vi "Update Bind Method Constants.vi"(7 "RPC Method Parameters":T1[](array[typedef]), 8 "error in (no error)":errorcluster, 10 "RPC Method Name":string, 11 "VI in":refnum<vi>) -> (0 "error out":errorcluster, 3 "VI out":refnum<vi>)   [LabVIEW 2019, in "gRPC Scripting Tools.lvlib"]
uses:
  gRPC Scripting Tools.lvlib
  TypeDefs/RPC Method Parameters.ctl
  <vilib>/Utility/traverseref.llb/TRef TravTarget.ctl
  <vilib>/Utility/traverseref.llb/VI Scripting - Traverse.lvlib
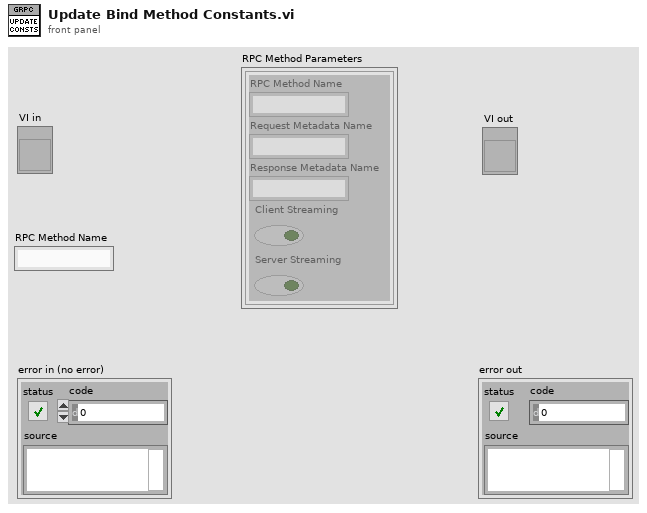
[diagram p1: front panel]
types:
  T1 = typedef "gRPC Scripting Tools.lvlib/RPC Method Parameters.ctl" = cluster{"RPC Method Name":string, "Request Metadata Name":string, "Response Metadata Name":string, "Client Streaming":bool, "Server Streaming":bool}
  T2 = typedef "TRef TravTarget.ctl" = enum16{"FP", "BD", "Other"}
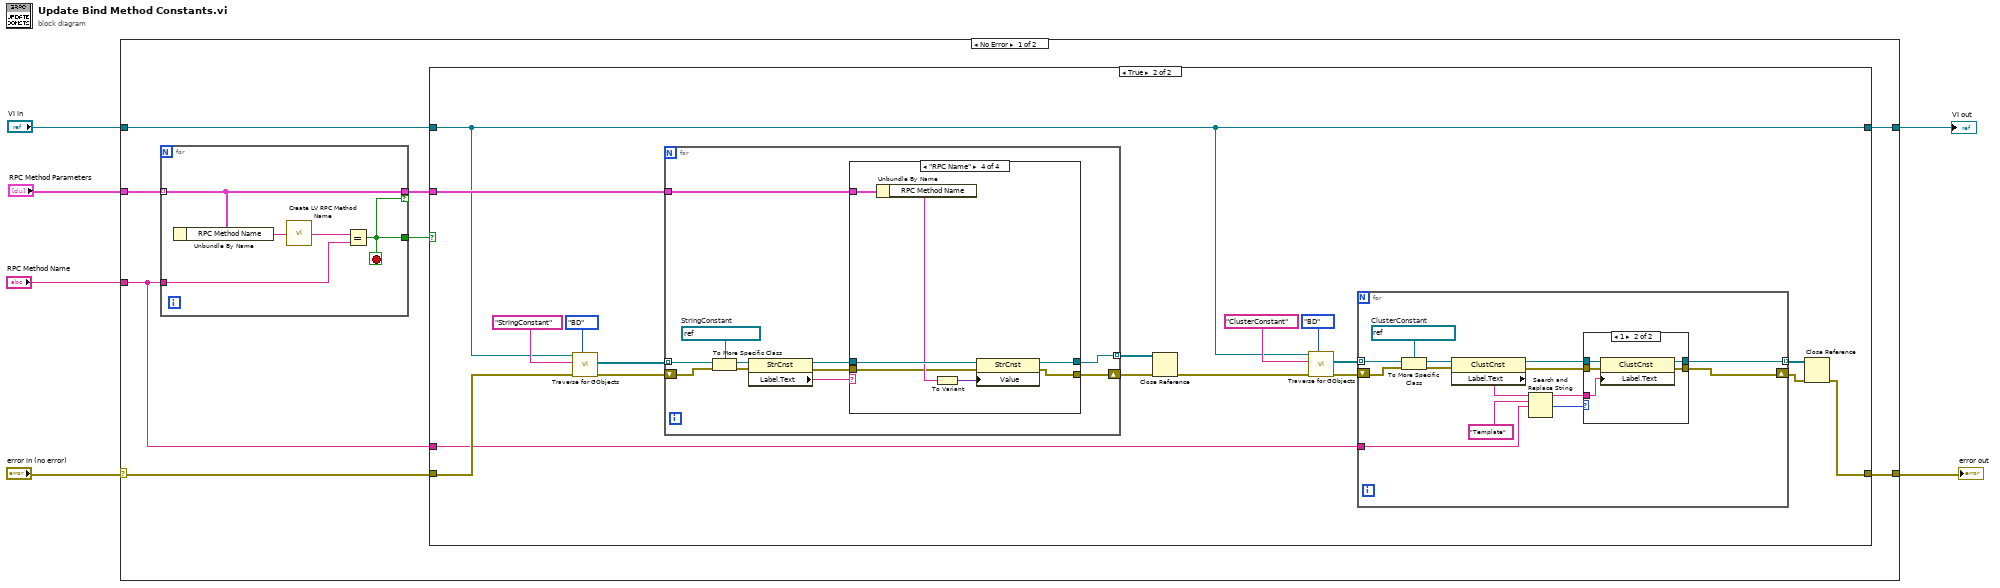
[diagram p0: block diagram]
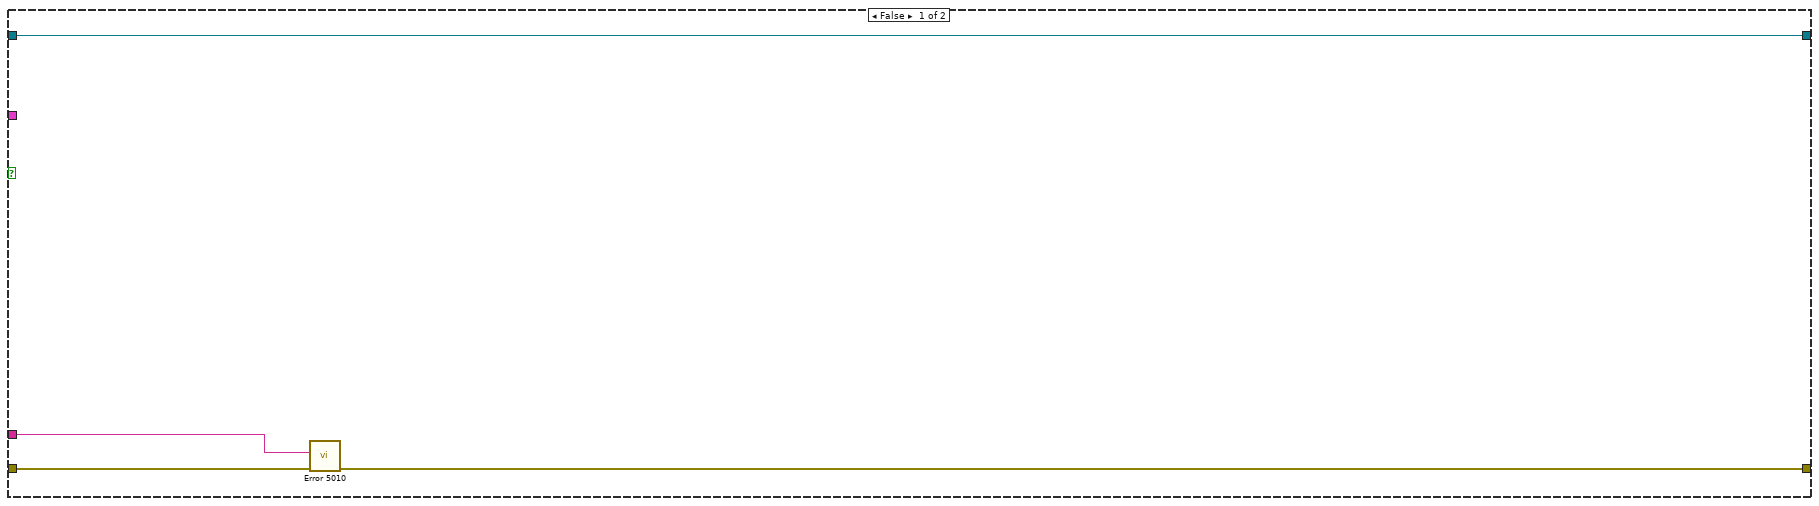
[diagram p2: hidden frame]
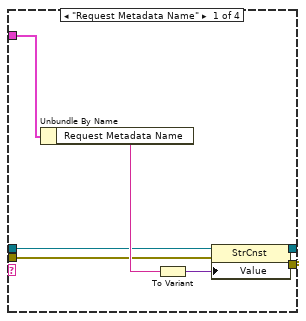
[diagram p4: hidden frame]
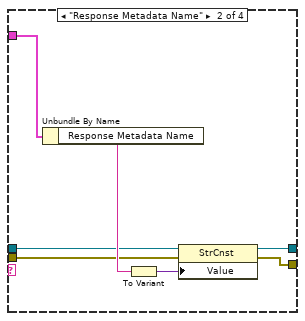
[diagram p5: hidden frame]
diagram:
  n1 = case shown="No Error" "error in (no error)" {
    selector: "error in (no error)" -> [w9 w98]
    tunnel: [w14 w98] -> w6
    tunnel: "VI in" -> [w13 w97]
    tunnel: "RPC Method Parameters" -> [w12 _]
    tunnel: "RPC Method Name" -> [w7 _]
    tunnel: [w8 w97] -> w1
    frame No Error {
      n2 = for {
        tunnel: w12 -> [w95] mode=indexing
        tunnel: w7 -> [w96]
        tunnel: [w95] -> w10 if=w94
        tunnel: [w94] -> w11
        stop <- w94 stop-if-true
        n3 = Unbundle By Name(w95) -> ("RPC Method Name"=w93:string)
        n4 = call "Create LV RPC Method Name.vi"("Proto Parser RPC Method Name in"=w93) -> ("LV RPC Method Name out"=w92:string)
        n5 = Equal?(x=w92, y=w96) -> (x = y?=w94:bool)
      }
      n6 = case shown="True" w11 {
        tunnel: [w15 w20] -> w14
        tunnel: w9 -> [w17 w36]
        tunnel: w13 -> [w18 w25]
        tunnel: w10 -> [_ w32]
        tunnel: [w18 w25] -> w8
        tunnel: w7 -> [w16 w22]
        frame False {
          n7 = call "Error 5010.vi"("error in (no error)"=w17, "RPC Method Name"=w16) -> ("error out"=w15:errorcluster)  [unwired: 9 in]
        }
        frame True {
          n8 = call <vilib>:"Traverse for GObjects.vi"("Traverse Target"=TRef_TravTarget."BD", "error in (no error)"=w36, "Class Name"="StringConstant", "VI Refnum"=w25) -> ("error out"=w33:errorcluster, "References"=w28:refnum<vi>[])  [unwired: 4 in, 2 out]
          n9 = for {
            tunnel: w28 -> [w67] mode=indexing
            shift-right: [w59] -> w29
            shift-left: w33 -> [w66]
            tunnel: w32 -> [w62]
            tunnel: [w58] -> w27 mode=indexing
            w68 = refnum<vi> refnum  # StringConstant
            n10 = To More Specific Class(target class=w68, reference=w67, error in=w66) -> (specific class reference=w65:refnum<vi>, error out=w64:errorcluster)
            n11 = property class="StrCnst"(reference=w65, error in=w64) -> (reference out=w61:refnum<vi>, error out=w60:errorcluster, "Label.Text"=w63:string)
            n12 = case shown="\"RPC Name\"" w63 {
              tunnel: w62 -> [w70 w80 _ w91]
              tunnel: w61 -> [w72 w78 w83 w90]
              tunnel: w60 -> [w73 w79 w84 w87]
              tunnel: [w71 w77 w84 w86] -> w59
              tunnel: [w69 w76 w83 w85] -> w58
              frame "Request Metadata Name" {
                n13 = Unbundle By Name(w70) -> ("Request Metadata Name"=w75:string)
                n14 = To Variant(anything=w75) -> (Variant=w74:variant)
                n15 = property class="StrCnst"(reference=w72, error in=w73, "Value"=w74) -> (reference out=w69:refnum<vi>, error out=w71:errorcluster)
              }
              frame "Response Metadata Name" {
                n16 = Unbundle By Name(w80) -> ("Response Metadata Name"=w82:string)
                n17 = To Variant(anything=w82) -> (Variant=w81:variant)
                n18 = property class="StrCnst"(reference=w78, error in=w79, "Value"=w81) -> (reference out=w76:refnum<vi>, error out=w77:errorcluster)
              }
              frame "None", Default {
              }
              frame "RPC Name" {
                n19 = Unbundle By Name(w91) -> ("RPC Method Name"=w89:string)
                n20 = To Variant(anything=w89) -> (Variant=w88:variant)
                n21 = property class="StrCnst"(reference=w90, error in=w87, "Value"=w88) -> (reference out=w85:refnum<vi>, error out=w86:errorcluster)
              }
            }
          }
          n22 = Close Reference(reference=w27, error in (no error)=w29) -> (error out=w26:errorcluster)
          n23 = call <vilib>:"Traverse for GObjects.vi"("Traverse Target"=TRef_TravTarget."BD", "error in (no error)"=w26, "Class Name"="ClusterConstant", "VI Refnum"=w25) -> ("error out"=w24:errorcluster, "References"=w23:refnum<vi>[])  [unwired: 4 in, 2 out]
          n24 = for {
            tunnel: w23 -> [w49] mode=indexing
            shift-right: [w38] -> w21
            shift-left: w24 -> [w48]
            tunnel: w22 -> [w43]
            tunnel: [w37] -> w19 mode=indexing
            w50 = refnum<vi> refnum  # ClusterConstant
            n25 = To More Specific Class(target class=w50, reference=w49, error in=w48) -> (specific class reference=w47:refnum<vi>, error out=w46:errorcluster)
            n26 = property class="ClustCnst"(reference=w47, error in=w46) -> (reference out=w42:refnum<vi>, error out=w41:errorcluster, "Label.Text"=w44:string)
            n27 = Search and Replace String(input string=w44, search string="Template", replace string=w43) -> (result string=w39:string, number of replacements=w40:i32)  [unwired: 5 in, 2 out]
            n28 = case shown="1" w40 {
              tunnel: w42 -> [w52 w57]
              tunnel: [w52 w56] -> w37
              tunnel: [w51 w55] -> w38
              tunnel: w41 -> [w51 w54]
              tunnel: w39 -> [_ w53]
              frame 0, Default {
              }
              frame 1 {
                n29 = property class="ClustCnst"(reference=w57, error in=w54, "Label.Text"=w53) -> (reference out=w56:refnum<vi>, error out=w55:errorcluster)
              }
            }
          }
          n30 = Close Reference(reference=w19, error in (no error)=w21) -> (error out=w20:errorcluster)
        }
      }
    }
    frame Error {
    }
  }
  "error out" <- w6
  "VI out" <- w1
